vi "MessageBase.getNamesAndValues.Helper.vi"(8 "error in (no error)":errorcluster, 10 "FIeldSpec":T1, 11 "MessageBase in":refnum<class "MessageBase.lvclass">) -> (0 "error out":errorcluster, 2 "Array":cluster{"Value":variant, "Text":string}[](array[cluster]), 3 "MessageBase out":refnum<class "MessageBase.lvclass">)   [LabVIEW 2022 SP3]
uses:
  MessageBase.lvclass
  FieldSpec.ctl
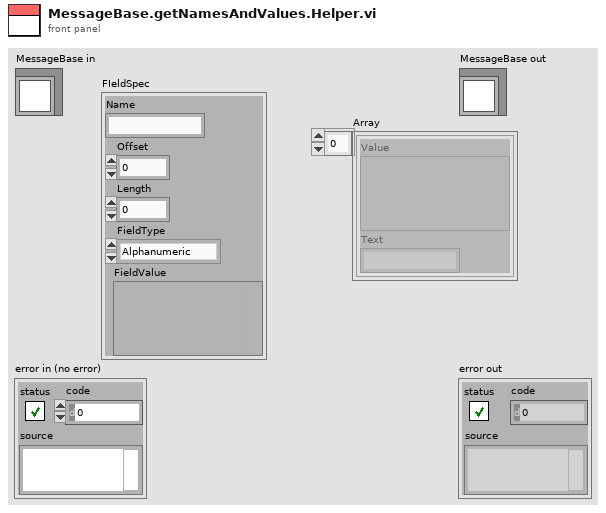
[diagram p1: front panel]
types:
  T1 = typedef "FieldSpec.ctl" = cluster{"Name":string, "Offset":i32, "Length":i32, "FieldType":enum16{"Alphanumeric", "Binary", "BinaryLongPrice", "BinaryShortPrice", "BitField", "PrintableAscii", "Value"}, "FieldValue":variant}
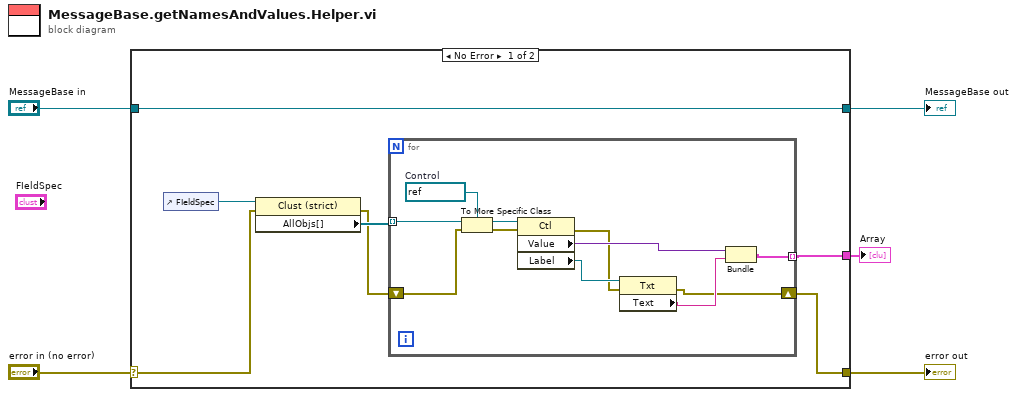
[diagram p0: block diagram]
diagram:
  n1 = case shown="No Error" "error in (no error)" {
    selector: "error in (no error)" -> [w10 w25]
    tunnel: [w6 w25] -> w4
    tunnel: [w12 w24] -> w2
    tunnel: "MessageBase in" -> [w12 w24]
    tunnel: [w7 _] -> w1
    frame No Error {
      n2 = control-ref of="FIeldSpec"() -> (w11:refnum<vi>)
      n3 = property class="Clust (strict)"(reference=w11, error in=w10) -> (error out=w8:errorcluster, "AllObjs[]"=w9:refnum<vi>[])  [unwired: 1 out]
      n4 = for {
        tunnel: w9 -> [w23] mode=indexing
        tunnel: [w16] -> w7 mode=indexing
        shift-right: [w13] -> w6
        shift-left: w8 -> [w15]
        w22 = refnum<vi> refnum  # Control
        n5 = To More Specific Class(target class=w22, reference=w23, error in=w15) -> (specific class reference=w21:refnum<vi>, error out=w20:errorcluster)
        n6 = property class="Ctl"(reference=w21, error in=w20) -> (error out=w14:errorcluster, "Value"=w19:variant, "Label"=w18:refnum<vi>)  [unwired: 1 out]
        n7 = property class="Txt"(reference=w18, error in=w14) -> (error out=w13:errorcluster, "Text"=w17:string)  [unwired: 1 out]
        n8 = Bundle("Value"=w19, "Text"=w17) -> (w16:cluster{"Value":variant, "Text":string})  [unwired: 1 in]
      }
    }
    frame Error {
    }
  }
  "error out" <- w4
  "MessageBase out" <- w2
  "Array" <- w1
